vi "svl_Check Decimation Factor.vi"(4 "decimation factor":i32=1 min=1 step=1, 6 "time constant [ms]":dbl=125.0 format="%.2f", 8 "error in (no error)":errorcluster, 9 "restart averaging (F)":bool, 10 "dt":dbl=125.0 format="%.2f") -> (0 "error out":errorcluster, 2 "parameter has changed":bool)   [LabVIEW 2017]
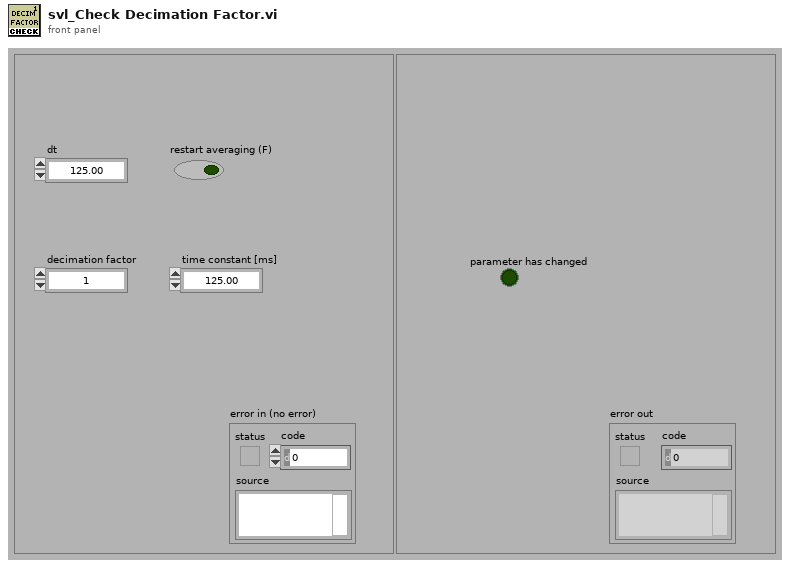
[diagram p1: front panel]
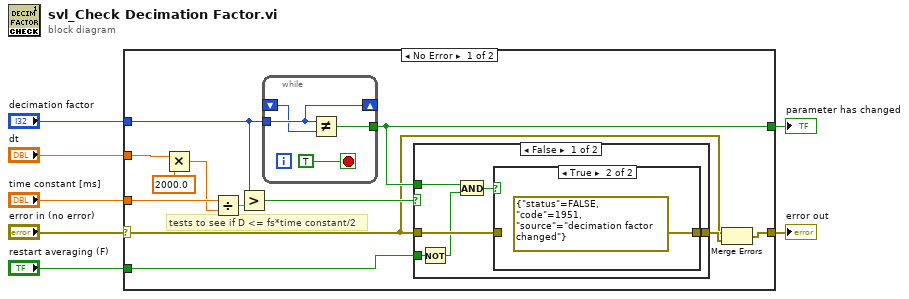
[diagram p0: block diagram]
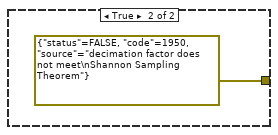
[diagram p3: hidden frame]
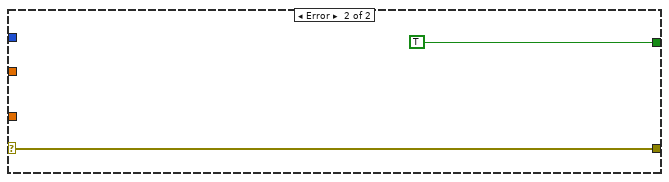
[diagram p4: hidden frame]
diagram:
  n1 = case shown="No Error" "error in (no error)" {
    selector: "error in (no error)" -> [w8 w33]
    tunnel: [w11 TRUE] -> w4
    tunnel: "decimation factor" -> [w15 _]
    tunnel: [w10 w33] -> w5
    tunnel: "time constant [ms]" -> [w19 _]
    tunnel: "dt" -> [w14 _]
    tunnel: "restart averaging (F)" -> [w12 _]
    frame No Error {
      # "tests to see if D <= fs*time constant/2"
      n2 = Multiply(x=w14, y=2000.0) -> (x*y=w17:dbl)
      n3 = Divide(x=w19, y=w17) -> (x/y=w16:dbl)
      n4 = Greater?(x=w15, y=w16) -> (0:w13:bool)
      n5 = while {
        tunnel: [w20] -> w11
        tunnel: w15 -> [w22]
        shift-left: _ -> [w21]
        shift-right: [w22] -> _
        stop <- TRUE stop-if-true
        n6 = Not Equal?(x=w22, y=w21) -> (x != y?=w20:bool)
      }
      n7 = case shown="False" w13 {
        tunnel: w8 -> [w29 _]
        tunnel: [w28 errorcluster {"status"=FALSE, "code"=1950, "source"="decimation factor does not meet\nShannon Sampling Theorem"} ("error IO")] -> w9
        tunnel: w12 -> [w27 _]
        tunnel: w11 -> [w25 _]
        frame False {
          n8 = Not(x=w27) -> (.not. x?=w24:bool)
          n9 = And(x=w25, y=w24) -> (x .and. y?=w26:bool)
          n10 = case shown="True" w26 {
            tunnel: w29 -> [w30 _]
            tunnel: [w30 errorcluster {"status"=FALSE, "code"=1951, "source"="decimation factor changed"} ("error IO")] -> w28
            frame False {
            }
            frame True {
            }
          }
        }
        frame True {
        }
      }
      n11 = Merge Errors(w8, w9) -> (w10:errorcluster)
    }
    frame Error {
    }
  }
  "parameter has changed" <- w4
  "error out" <- w5
